vi "Multiplication9225-7_FPGA.vi"(1 "y <+/-44,8>":fxp<+/-,44,8>, 2 "x <+/-47,6>":fxp<+/-,47,6>) -> (0 "x*y <+/-49,13>":fxp<+/-,49,13>)   [LabVIEW 2021]
uses:
  <vilib>/rvi/FXPMathLib/FxpMul/XNode/nifxpmath_Multiplier.xnode
  <vilib>/rvi/FXPMathLib/sim/FxpSim.dll
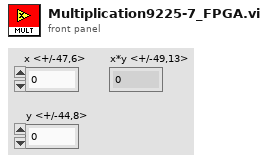
[diagram p1: front panel]
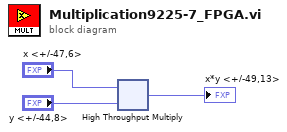
[diagram p0: block diagram]
diagram:
  n1 = xnode "High Throughput Multiply"("x"="x <+/-47,6>", "y"="y <+/-44,8>") -> ("x*y"=→"x*y <+/-49,13>":fxp<+/-,49,13>)
